vi "ParseAgentMessage.vi"(8 "Error In":errorcluster, 9 "AgentMessage":T5, 10 "SessionId":string, 11 "LiteAgent In":T1) -> (0 "Error Out":errorcluster, 1 "Completions":T3, 2 "Content":T2, 3 "LiteAgent Out":T1, 5 "Common":T4)   [LabVIEW 2017]
uses:
  C:/Users/Jan/Projects/LiteAgentSDK-LabVIEW/Source/Bin/LiteAgentSDK.LabVIEW.dll
  Bin/LiteAgentSDK.LabVIEW.dll
  <vilib>/LVH/i3 JSON/JSON Parsing/Get Array Value at Index Files/Get Array Value at Index - Object.vi
  <vilib>/LVH/i3 JSON/i3-json.lvlib
  <vilib>/addons/Tools/Unicode/UTF8 Tools.lvlib
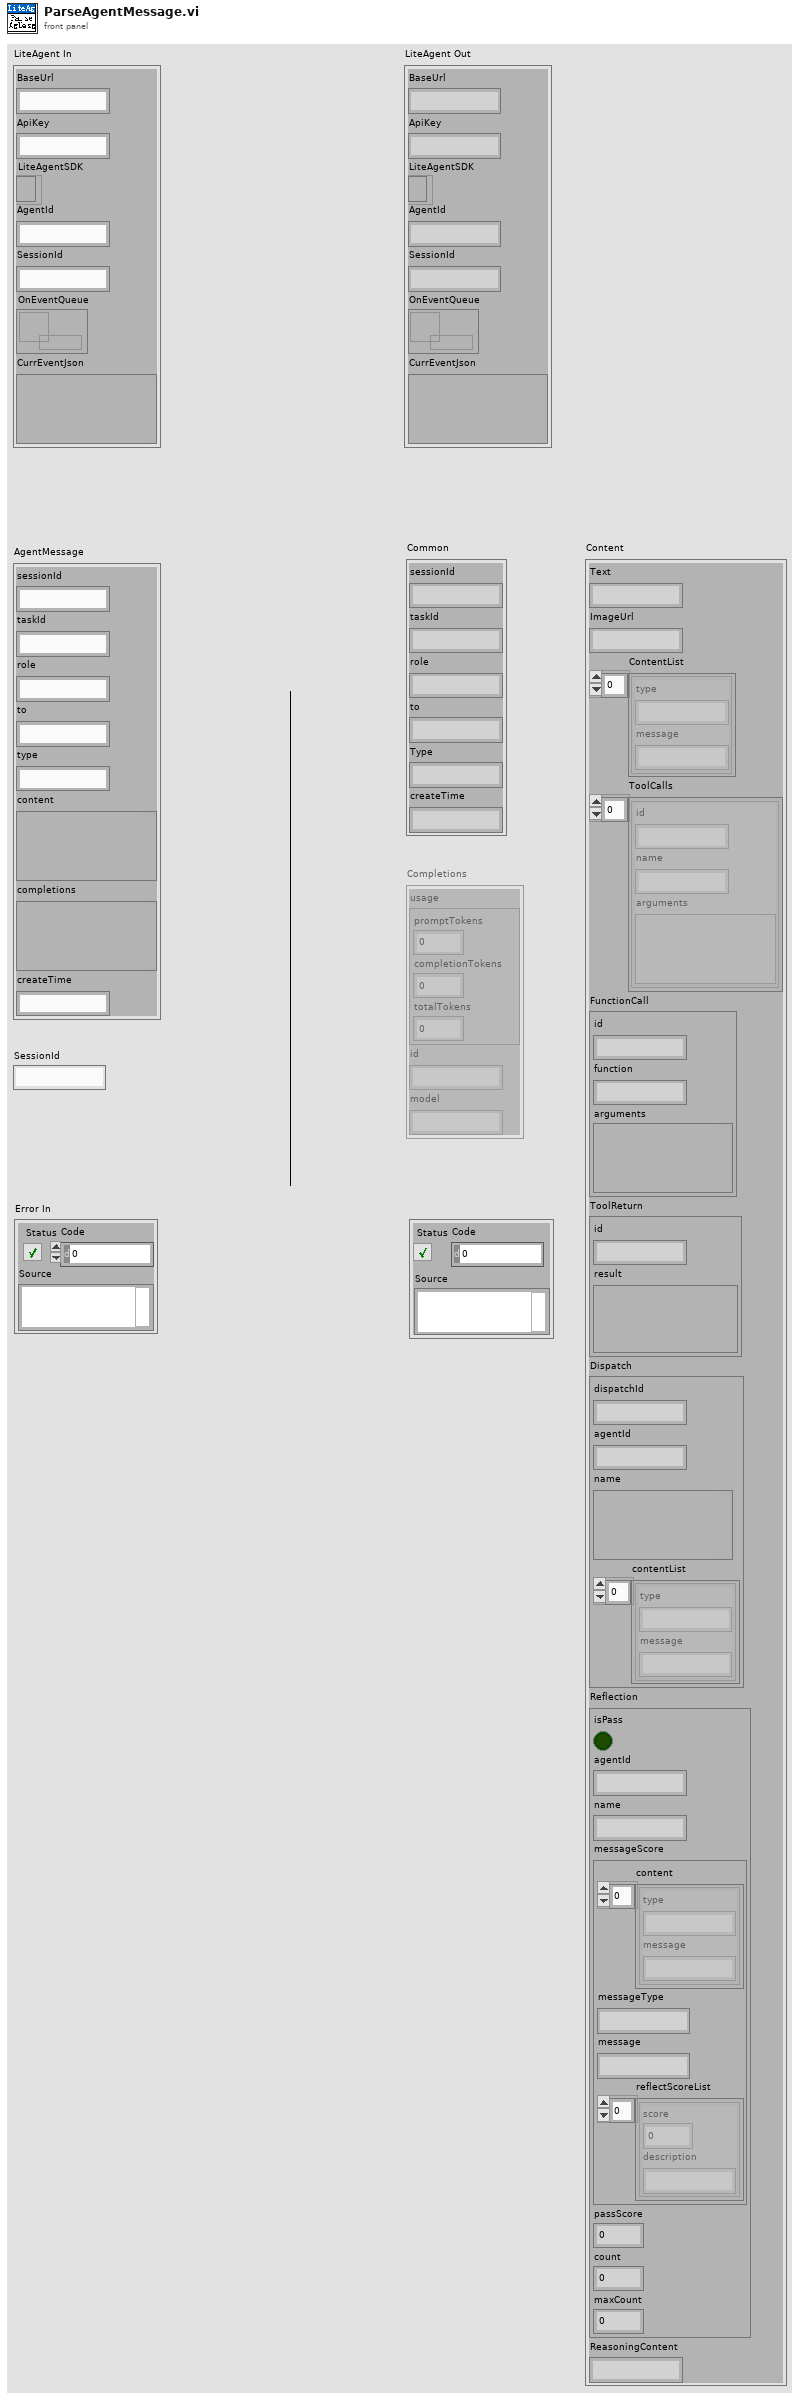
[diagram p1: front panel]
types:
  T1 = cluster{"BaseUrl":string, "ApiKey":string, "LiteAgentSDK":refnum<k24>, "AgentId":string, "SessionId":string, "OnEventQueue":refnum<queue>, "CurrEventJson":variant}
  T2 = cluster{"Text":string, "ImageUrl":string, "ContentList":cluster{"type":string, "message":string}[], "ToolCalls":cluster{"id":string, "name":string, "arguments":variant}[], "FunctionCall":cluster{"id":string, "function":string, "arguments":variant}, "ToolReturn":cluster{"id":string, "result":variant}, "Dispatch":cluster{"dispatchId":string, "agentId":string, "name":variant, "contentList":cluster{"type":string, "message":string}[]}, "Reflection":cluster{"isPass":bool, "agentId":string, "name":string, "messageScore":cluster{"content":cluster{"type":string, "message":string}[], "messageType":string, "message":string, "reflectScoreList":cluster{"score":i32, "description":string}[]}, "passScore":i32, "count":i32, "maxCount":i32}, "ReasoningContent":string}
  T3 = cluster{"usage":cluster{"promptTokens":i32, "completionTokens":i32, "totalTokens":i32}, "id":string, "model":string}
  T4 = cluster{"sessionId":string, "taskId":string, "role":string, "to":string, "Type":string, "createTime":string}
  T5 = cluster{"sessionId":string, "taskId":string, "role":string, "to":string, "type":string, "content":variant, "completions":variant, "createTime":string}
  T6 = enum8{"Enabled", "Disabled", "Disabled and Grayed Out"}
  T7 = cluster{"id":string, "name":string, "arguments":variant}
  T8 = cluster{"id":string, "function":string, "arguments":variant}
  T9 = cluster{"dispatchId":string, "agentId":string, "name":variant, "contentList":cluster{"type":string, "message":string}[]}
  T10 = cluster{"isPass":bool, "agentId":string, "name":string, "messageScore":cluster{"content":cluster{"type":string, "message":string}[], "messageType":string, "message":string, "reflectScoreList":cluster{"score":i32, "description":string}[]}, "passScore":i32, "count":i32, "maxCount":i32}
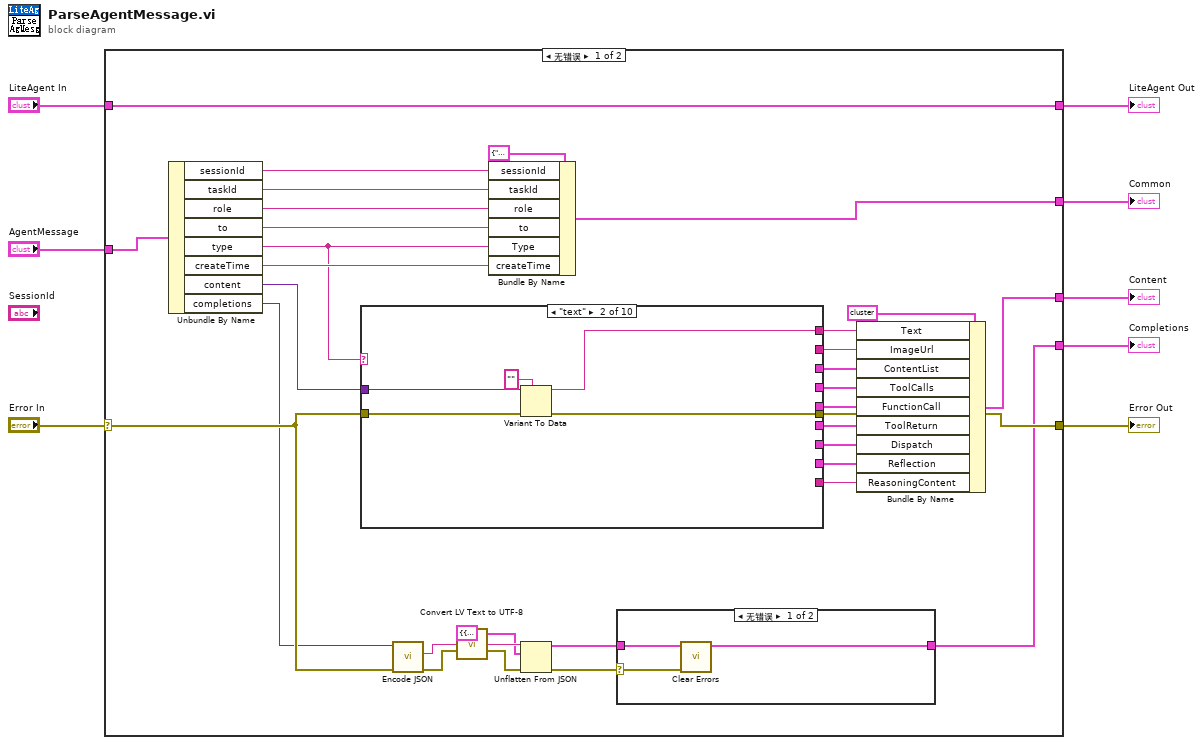
[diagram p0: block diagram]
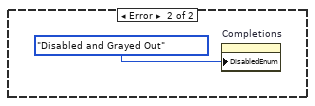
[diagram p2: hidden frame]
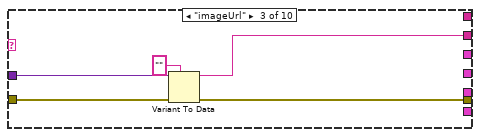
[diagram p4: hidden frame]
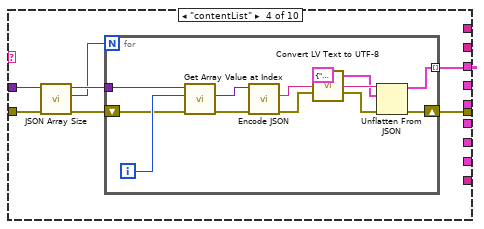
[diagram p5: hidden frame]
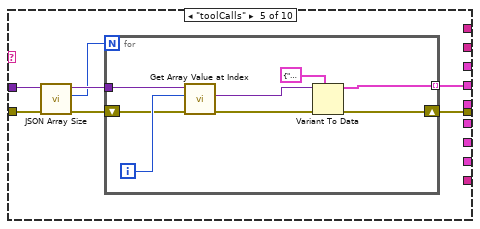
[diagram p6: hidden frame]
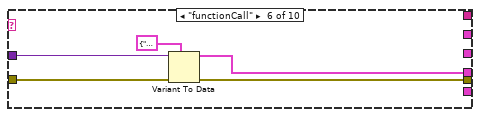
[diagram p7: hidden frame]
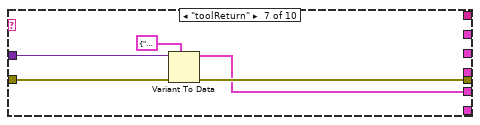
[diagram p8: hidden frame]
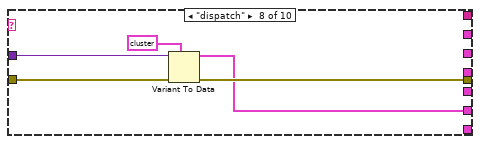
[diagram p9: hidden frame]
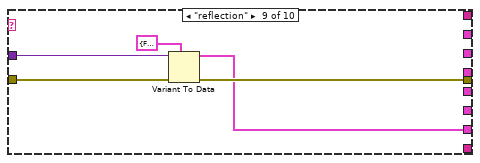
[diagram p10: hidden frame]
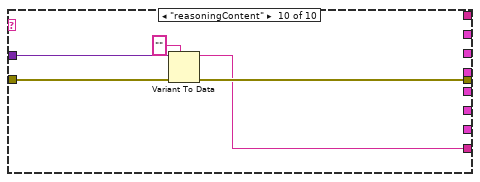
[diagram p11: hidden frame]
diagram:
  n1 = case shown="无错误" "Error In" {
    selector: "Error In" -> [w13 w116]
    tunnel: [w19 w116] -> w7
    tunnel: "AgentMessage" -> [w41 _]
    tunnel: [w36 _] -> w3
    tunnel: [w24 _] -> w5
    tunnel: [w11 _] -> w4
    tunnel: "LiteAgent In" -> [w20 w115]
    tunnel: [w20 w115] -> w1
    frame No Error {
      n2 = Unbundle By Name(w41) -> ("sessionId"=w40:string, "taskId"=w39:string, "role"=w38:string, "to"=w37:string, "type"=w21:string, "createTime"=w22:string, "content"=w34:variant, "completions"=w12:variant)
      n3 = case shown="\"text\"" w21 {
        tunnel: w34 -> [_ w50 w53 w58 w77 w91 w97 w102 w107 w110]
        tunnel: w13 -> [w45 w49 w54 w59 w78 w94 w99 w104 w109 w113]
        tunnel: [w45 w48 w52 w56 w75 w93 w98 w103 w108 w112] -> w19
        tunnel: [_ w46 _ _ _ _ _ _ _ _] -> w33
        tunnel: [_ _ w51 _ _ _ _ _ _ _] -> w32
        tunnel: [_ _ _ w57 _ _ _ _ _ _] -> w31
        tunnel: [_ _ _ _ w76 _ _ _ _ _] -> w30
        tunnel: [_ _ _ _ _ w90 _ _ _ _] -> w29
        tunnel: [_ _ _ _ _ _ w95 _ _ _] -> w28
        tunnel: [_ _ _ _ _ _ _ w100 _ _] -> w27
        tunnel: [_ _ _ _ _ _ _ _ w105 _] -> w26
        tunnel: [_ _ _ _ _ _ _ _ _ w111] -> w25
        frame "", Default {
        }
        frame "text" {
          n4 = Variant To Data(error in=w49, type="", Variant=w50) -> (data=w46:string, error out=w48:errorcluster)
        }
        frame "imageUrl" {
          n5 = Variant To Data(error in=w54, type="", Variant=w53) -> (data=w51:string, error out=w52:errorcluster)
        }
        frame "contentList" {
          n6 = call <vilib>:"JSON Array Size.vi"("error in (no error)"=w59, "JSON Tree In (JSON Array)"=w58) -> ("error out"=w62:errorcluster, "Array Size"=w60:i32, "JSON Tree Passthrough (JSON Array)"=w61:variant)  [unwired: 7 in]
          n7 = for {
            N: w60 -> [_]
            shift-right: [w65] -> w56
            shift-left: w62 -> [w72]
            tunnel: [w63] -> w57 mode=indexing
            tunnel: w61 -> [w74]
            i -> [w73]
            n8 = call-poly <vilib>:"Get Array Value at Index.vi"("error in (no error)"=w72, "Index"=w73, "JSON Tree In (JSON Array)"=w74) -> ("error out"=w66:errorcluster, "JSON Object"=w67:variant)  [unwired: 5 in, 2 out]
            n9 = call <vilib>:"Encode JSON.vi"("error in (no error)"=w66, "JSON Tree"=w67) -> ("error out"=w71:errorcluster, "String"=w68:string)  [unwired: 4 in]
            n10 = call <vilib>:"Convert LV Text to UTF-8.vi"("LV Text"=w68, "error in"=w71) -> ("UTF-8 Text"=w69:string, "error out"=w70:errorcluster)  [unwired: 12 in]
            n11 = Unflatten From JSON(JSON string=w69, type and defaults=cluster{"type":string, "message":string} {"type"="", "message"=""} ("Content"), error in (no error)=w70) -> (value=w63:cluster{"type":string, "message":string}, error out=w65:errorcluster)  [unwired: 4 in]
          }
        }
        frame "toolCalls" {
          n12 = call <vilib>:"JSON Array Size.vi"("error in (no error)"=w78, "JSON Tree In (JSON Array)"=w77) -> ("error out"=w81:errorcluster, "Array Size"=w79:i32, "JSON Tree Passthrough (JSON Array)"=w80:variant)  [unwired: 7 in]
          n13 = for {
            N: w79 -> [_]
            shift-right: [w85] -> w75
            shift-left: w81 -> [w87]
            tunnel: [w83] -> w76 mode=indexing
            tunnel: w80 -> [w89]
            i -> [w88]
            n14 = call-poly <vilib>:"Get Array Value at Index.vi"("error in (no error)"=w87, "Index"=w88, "JSON Tree In (JSON Array)"=w89) -> ("error out"=w86:errorcluster, "JSON Object"=w84:variant)  [unwired: 5 in, 2 out]
            n15 = Variant To Data(error in=w86, type=T7 {"id"="", "name"="", "arguments"=variant} ("ToolCall"), Variant=w84) -> (data=w83:T7, error out=w85:errorcluster)
          }
        }
        frame "functionCall" {
          n16 = Variant To Data(error in=w94, type=T8 {"id"="", "function"="", "arguments"=variant} ("FunctionCall"), Variant=w91) -> (data=w90:T8, error out=w93:errorcluster)
        }
        frame "toolReturn" {
          n17 = Variant To Data(error in=w99, type=cluster{"id":string, "result":variant} {"id"="", "result"=variant} ("ToolReturn"), Variant=w97) -> (data=w95:cluster{"id":string, "result":variant}, error out=w98:errorcluster)
        }
        frame "dispatch" {
          n18 = Variant To Data(error in=w104, type=T9 {"dispatchId"="", "agentId"="", "name"=variant, "contentList"=[]} ("Dispatch"), Variant=w102) -> (data=w100:T9, error out=w103:errorcluster)
        }
        frame "reflection" {
          n19 = Variant To Data(error in=w109, type=T10 {"isPass"=FALSE, "agentId"="", "name"="", "messageScore"={"content"=[], "messageType"="", "message"="", "reflectScoreList"=[]}, "passScore"=0, "count"=0, "maxCount"=0} ("Reflection"), Variant=w107) -> (data=w105:T10, error out=w108:errorcluster)
        }
        frame "reasoningContent" {
          n20 = Variant To Data(error in=w113, type="", Variant=w110) -> (data=w111:string, error out=w112:errorcluster)
        }
      }
      n21 = call <vilib>:"Encode JSON.vi"("error in (no error)"=w13, "JSON Tree"=w12) -> ("error out"=w18:errorcluster, "String"=w15:string)  [unwired: 4 in]
      n22 = call <vilib>:"Convert LV Text to UTF-8.vi"("LV Text"=w15, "error in"=w18) -> ("UTF-8 Text"=w16:string, "error out"=w17:errorcluster)  [unwired: 12 in]
      n23 = Bundle By Name(cluster=T4 {"sessionId"="", "taskId"="", "role"="", "to"="", "Type"="", "createTime"=""} ("Common"), "sessionId"=w40, "taskId"=w39, "role"=w38, "to"=w37, "Type"=w21, "createTime"=w22) -> (w36:T4)
      n24 = Unflatten From JSON(JSON string=w16, type and defaults=T3 {"usage"={"promptTokens"=0, "completionTokens"=0, "totalTokens"=0}, "id"="", "model"=""} ("Completions"), error in (no error)=w17) -> (value=w10:T3, error out=w9:errorcluster)  [unwired: 4 in]
      n25 = case shown="无错误" w9 {
        selector: w9 -> [w42 _]
        tunnel: w10 -> [w43 _]
        tunnel: [w43 _] -> w11
        frame No Error {
          n26 = call <vilib>:"Clear Errors.vi"("error in (no error)"=w42) -> ()  [unwired: 5 in, 2 out]
        }
        frame Error {
          n27 = property on="Completions" class="Clust (严格)"("DisabledEnum"=T6."Disabled and Grayed Out" ("禁用")) -> ()  [unwired: 2 in, 2 out]
        }
      }
      n28 = Bundle By Name(cluster=T2 {"Text"="", "ImageUrl"="", "ContentList"=[], "ToolCalls"=[], "FunctionCall"={"id"="", "function"="", "arguments"=variant}, "ToolReturn"={"id"="", "result"=variant}, "Dispatch"={"dispatchId"="", "agentId"="", "name"=variant, "contentList"=[]}, "Reflection"={"isPass"=FALSE, "agentId"="", "name"="", "messageScore"={"content"=[], "messageType"="", "message"="", "reflectScoreList"=[]}, "passScore"=0, "count"=0, "maxCount"=0}, "ReasoningContent"=""} ("Content"), "Text"=w33, "ImageUrl"=w32, "ContentList"=w31, "ToolCalls"=w30, "FunctionCall"=w29, "ToolReturn"=w28, "Dispatch"=w27, "Reflection"=w26, "ReasoningContent"=w25) -> (w24:T2)
    }
    frame Error {
    }
  }
  "Error Out" <- w7
  "Common" <- w3
  "Completions" <- w4
  "Content" <- w5
  "LiteAgent Out" <- w1
